vi "cw_2_4.vi"() -> ()   [LabVIEW 2022 SP3]
panel:
  out "seconds counted":dbl
  in  "stop":bool
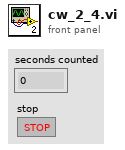
[diagram p1: front panel]
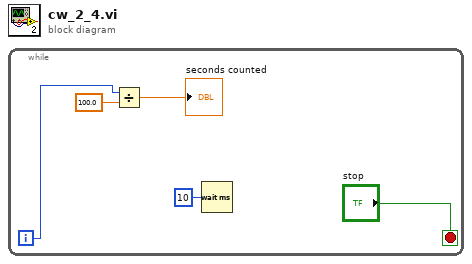
[diagram p0: block diagram]
diagram:
  n1 = while {
    i -> [w1]
    stop <- "stop" stop-if-true
    n2 = Divide(x=w1, y=100.0) -> (x/y=→"seconds counted":dbl)
    n3 = Wait (ms)(milliseconds to wait=u32 10) -> ()  [unwired: 1 out]
  }
